vi "test get_schemas.vi"() -> ()   [LabVIEW 2017]
uses:
  Database.lvlib
panel:
  out "Schemas":string[](array[string])
  in  "port":i32=33060
  in  "host":string="localhost"
  in  "password":string="carriker"
  in  "username":string="root"
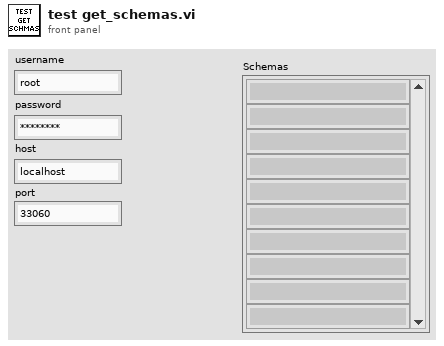
[diagram p1: front panel]
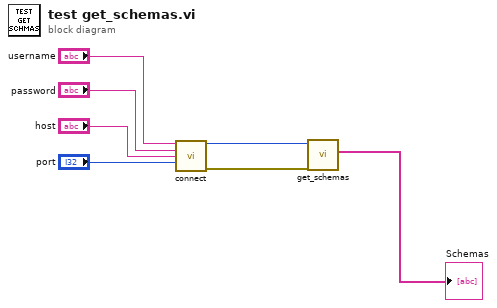
[diagram p0: block diagram]
diagram:
  n1 = call "connect.vi"("username"="username", "password"="password", "host"="host", "port"="port") -> ("DB Session ID"=w3:i32, "error out"=w2:errorcluster)  [unwired: 10 in]
  n2 = call "get_schemas.vi"("error in (no error)"=w2, "DB Session ID"=w3) -> ("Schemas"=→"Schemas":string[])  [unwired: 7 in, 2 out]
